vi "숫자형 배열.vi"() -> ()   [LabVIEW 2020]
panel:
  out "최소 인덱스":i32
  out "최솟값":dbl
  out "최대 인덱스":i32
  out "최대값":dbl
  out "두번째 부분 배열":dbl[](array[numeric])
  out "뒤집힌 배열":dbl[](array[numeric])
  out "첫번째 부분 배열":dbl[](array[numeric])
  out "원소의 인덱스":i32
  out "정렬된 배열":dbl[](array[numeric])
  in  "Array":dbl[](array[numeric])
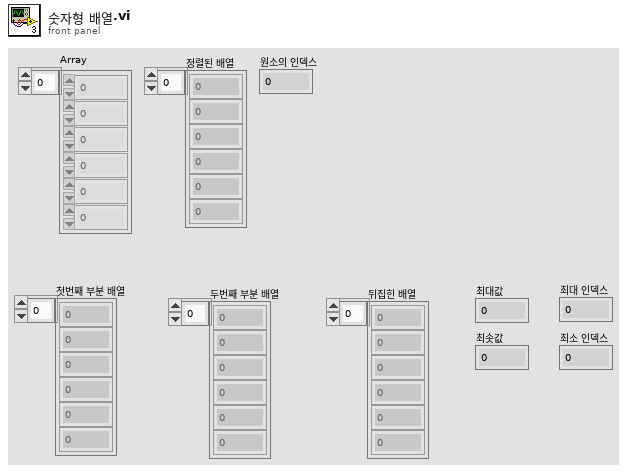
[diagram p1: front panel]
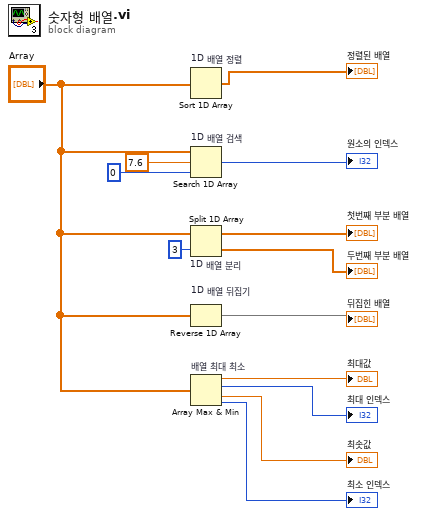
[diagram p0: block diagram]
diagram:
  n1 = Sort 1D Array "1D 배열 정렬"(array="Array") -> (sorted array=→"정렬된 배열":dbl[])
  n2 = Search 1D Array "1D 배열 검색"(1D array="Array", element=7.6, start index (0)=0) -> (index of element=→"원소의 인덱스":i32)
  n3 = Split 1D Array "1D 배열 분리"(array="Array", index=3) -> (first subarray=→"첫번째 부분 배열":dbl[], second subarray=→"두번째 부분 배열":dbl[])
  n4 = Reverse 1D Array "1D 배열 뒤집기"(array="Array") -> (reversed array=→"뒤집힌 배열":dbl[])
  n5 = Array Max & Min "배열 최대 최소"(array="Array") -> (max value=→"최대값":dbl, max index (indices)=→"최대 인덱스":i32, min value=→"최솟값":dbl, min index (indices)=→"최소 인덱스":i32)
